vi "frequency_sweep_modulation_freq_smooth.vi"(0 "Frequency":dbl, 1 "Channel (1:Channel 1)":i32, 2 "Amplitude (1.0 Vpp)":dbl=1.0 min=0.001 max=20.0 step=1.0 format="%#.3f", 3 "DC Offset (0.00 V)":dbl min=-10.0 max=10.0, 4 "SG Device 2":T1(ring) caption="Signal Generator Device", 5 "Modulation frequency":dbl[](array[numeric]), 6 "Current Sweep Value":refnum<vi>, 7 "Delay":dbl, 8 "Start t":refnum<vi>, 9 "Modulation Depth (0.0 %)":dbl, 11 "error in (no error)":errorcluster, 12 "Siglent Name":refnum<visa-resource-name>="USB0::0xF4EC::0x1102::SDG2XCAD4R3627::INSTR", 13 "AD2 2":i32, 14 "Stop 2":bool) -> (15 "error out":errorcluster)   [LabVIEW 2024, in "Sweep.lvlib"]
uses:
  Sweep.lvlib
  AD2/Node Parameters.ctl
  <instrlib>/Siglent SDG 1000 5000 800 Series/Public/Configure/Configure Modulation (AM).vi
  <instrlib>/Siglent SDG 1000 5000 800 Series/Siglent SDG 1000 5000 800 Series.lvlib
  AD2/AD2 DLL.lvlib
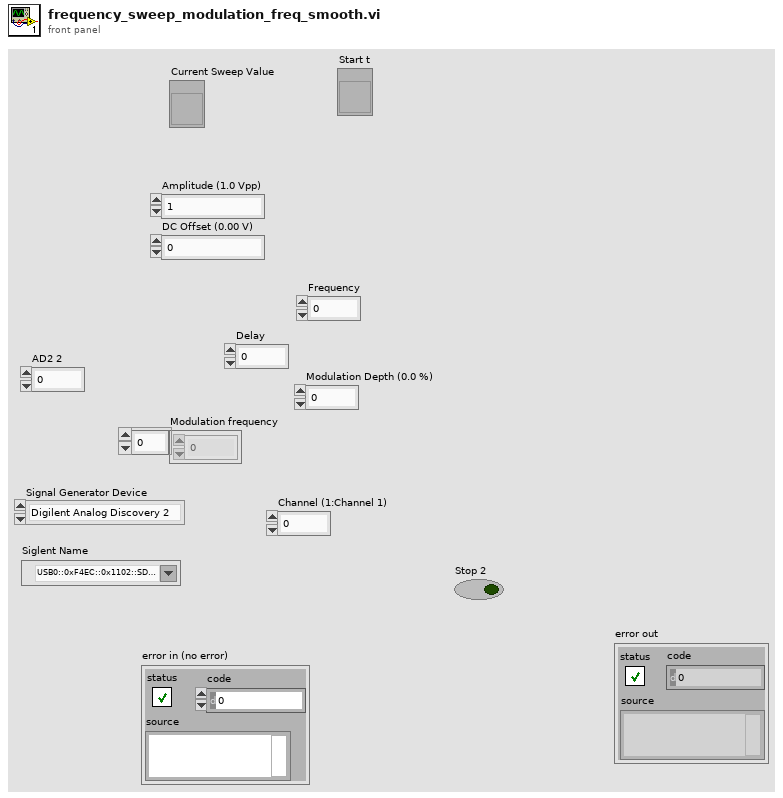
[diagram p1: front panel]
types:
  T1 = enum16{"Digilent Analog Discovery 2", "Siglent DG"}
  T2 = typedef "AD2 DLL.lvlib/Node Parameters.ctl" = cluster{"Function":u8, "Frequency":dbl, "Amplitude":dbl, "DC Offset":dbl, "Duty Cycle":dbl, "Phase":dbl}
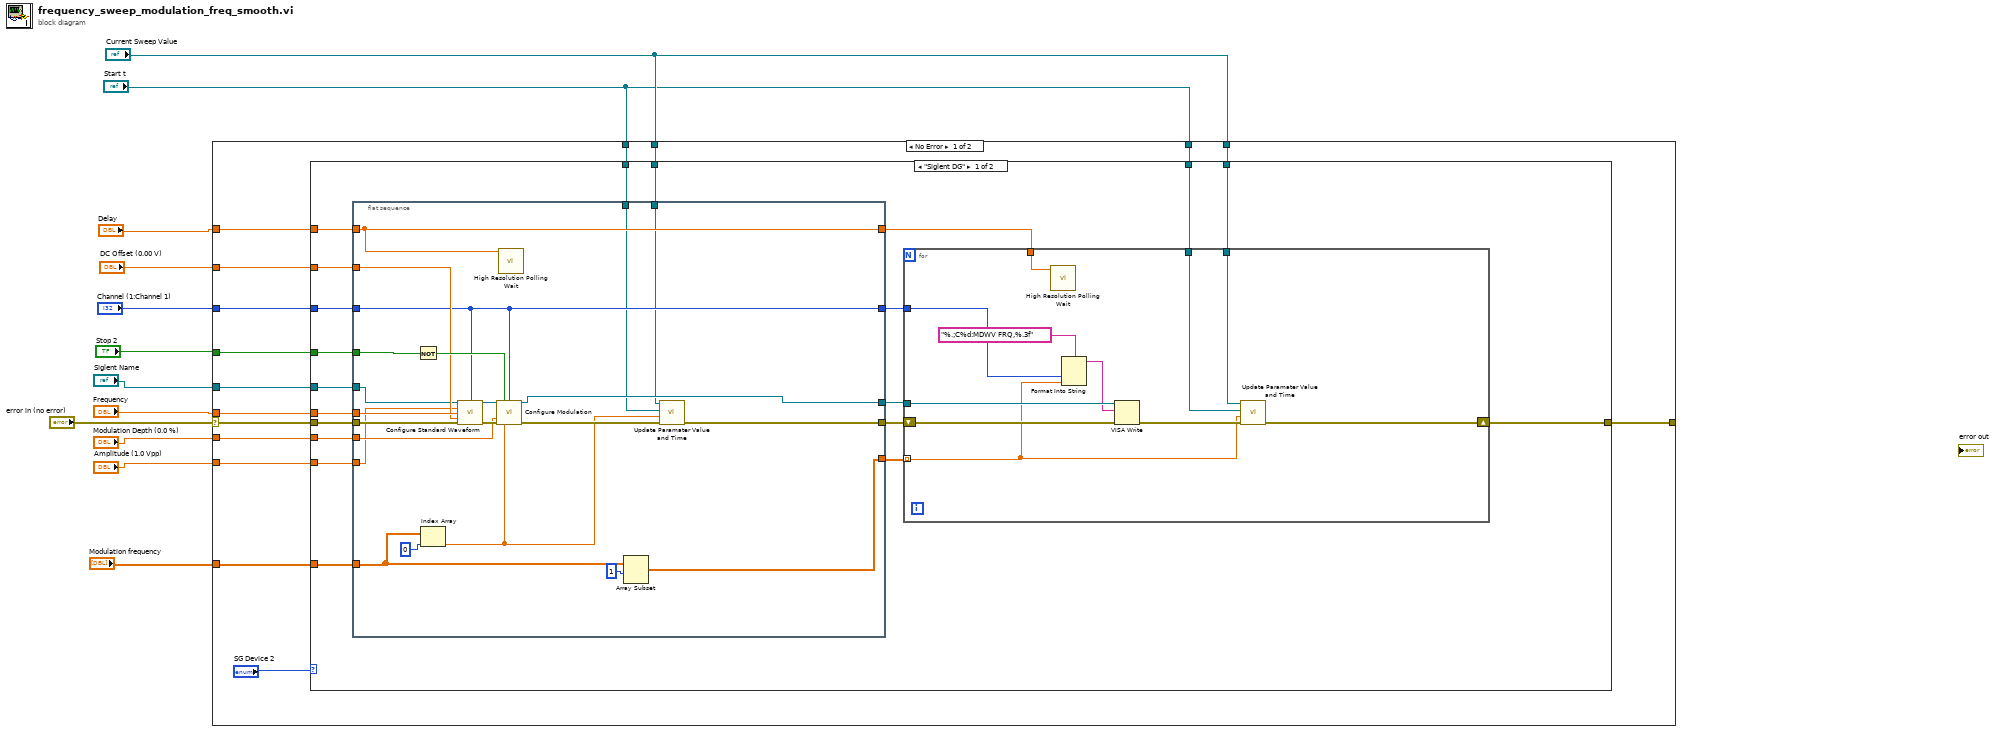
[diagram p0: block diagram]
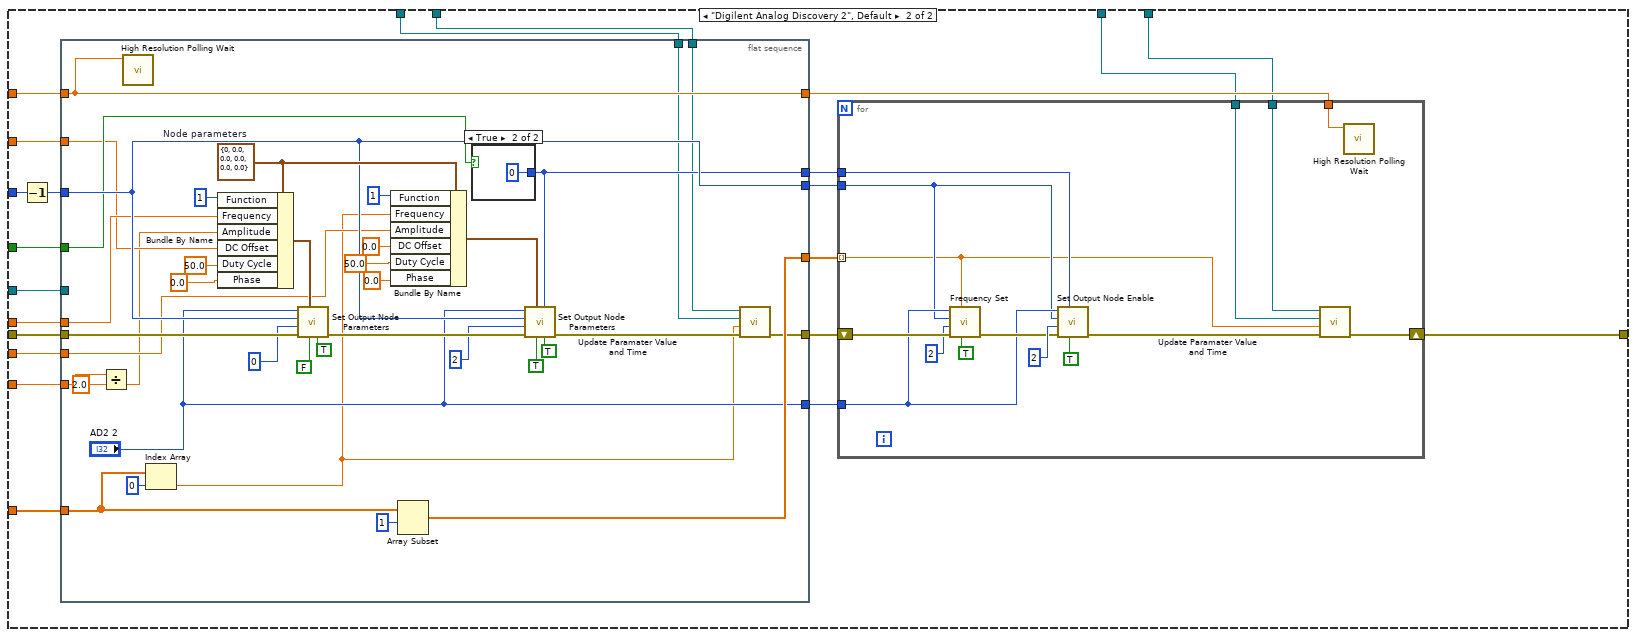
[diagram p2: hidden frame]
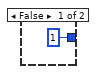
[diagram p3: hidden frame]
diagram:
  n1 = case shown="No Error" "error in (no error)" {
    selector: "error in (no error)" -> [w18 w159]
    tunnel: "Modulation Depth (0.0 %)" -> [w28 _]
    tunnel: "Amplitude (1.0 Vpp)" -> [w27 _]
    tunnel: "Frequency" -> [w26 _]
    tunnel: "Stop 2" -> [w25 _]
    tunnel: [w24 w159] -> _
    tunnel: "Modulation frequency" -> [w23 _]
    tunnel: "Channel (1:Channel 1)" -> [w22 _]
    tunnel: "Delay" -> [w21 _]
    tunnel: "DC Offset (0.00 V)" -> [w20 _]
    tunnel: "Siglent Name" -> [w19 _]
    tunnel: "Current Sweep Value" -> [w16 _]
    tunnel: "Current Sweep Value" -> [w15 _]
    tunnel: "Start t" -> [w14 _]
    tunnel: "Start t" -> [w13 _]
    frame No Error {
      n2 = case shown="\"Siglent DG\"" "SG Device 2" {
        tunnel: w28 -> [w47 w103]
        tunnel: w27 -> [w46 w102]
        tunnel: w26 -> [w45 w101]
        tunnel: w25 -> [w44 w100]
        tunnel: [w42 w98] -> w24
        tunnel: w23 -> [w41 w97]
        tunnel: w22 -> [w39 w95]
        tunnel: w21 -> [w38 w94]
        tunnel: w20 -> [w37 w93]
        tunnel: w19 -> [w36 w92]
        tunnel: w18 -> [w35 w91]
        tunnel: w16 -> [w32 w85]
        tunnel: w15 -> [w31 w84]
        tunnel: w14 -> [w30 w83]
        tunnel: w13 -> [w29 w82]
        frame "Siglent DG" {
          n3 = flat-sequence {
            tunnel: [w69] -> w48
            tunnel: w47 -> [w66]
            tunnel: w46 -> [w54]
            tunnel: w45 -> [w65]
            tunnel: w44 -> [w64]
            tunnel: [w52] -> w43
            tunnel: w41 -> [w62]
            tunnel: [w60] -> w40
            tunnel: w39 -> [w55]
            tunnel: w38 -> [w56]
            tunnel: w37 -> [w59]
            tunnel: w36 -> [w58]
            tunnel: w35 -> [w57]
            tunnel: [w56] -> w34
            tunnel: [w55] -> w33
            tunnel: w32 -> [w49]
            tunnel: w30 -> [w50]
            frame #0 {
              n4 = Not(x=w64) -> (.not. x?=w70:bool)
              n5 = Index Array(array=w62, index=0) -> (element=w51:dbl)
              n6 = call <instrlib>:"Configure Standard Waveform.vi"("VISA resource name"=w58, "Channel (1:Channel 1)"=w55, "Amplitude (1.0 Vpp)"=w54, "Frequency (1000 Hz)"=w65, "DC Offset (0.00 V)"=w59, "error in (no error)"=w57) -> ("VISA resource name out"=w67:refnum<visa-resource-name>, "error out"=w68:errorcluster)  [unwired: 8 in]
              n7 = call-poly <instrlib>:"Configure Modulation.vi"("VISA resource name"=w67, "Enable Amplitude Modulation (T:Enable)"=w70, "Channel (1:Channel 1)"=w55, "Modulation Depth (0.0 %)"=w66, "error in (no error)"=w68, "Modulation Frequency (100 Hz)"=w51) -> ("VISA resource name out"=w69:refnum<visa-resource-name>, "error out"=w53:errorcluster)  [unwired: 8 in]
              n8 = call <vilib>:"High Resolution Polling Wait.vi"("seconds to wait"=w56) -> ()  [unwired: 10 in, 1 out]
              n9 = Array Subset "Array Subset"(array=w62, index=1) -> (w60:dbl[])  [unwired: 1 in]
              n10 = call "Update Paramater Value and Time.vi"("error in (no error)"=w53, "Value"=w51, "Start t"=w50, "Current Sweep Value"=w49) -> ("error out"=w52:errorcluster)  [unwired: 7 in]
            }
          }
          n11 = for {
            shift-right: [w74] -> w42
            shift-left: w43 -> [w77]
            tunnel: w48 -> [w79]
            tunnel: w34 -> [w76]
            tunnel: w40 -> [w73] mode=indexing
            tunnel: w33 -> [w81]
            tunnel: w31 -> [w72]
            tunnel: w29 -> [w71]
            n12 = call <vilib>:"High Resolution Polling Wait.vi"("seconds to wait"=w76) -> ()  [unwired: 10 in, 1 out]
            n13 = Format Into String(format string="%.;C%d:MDWV FRQ,%.3f", w81, w73) -> (resulting string=w78:string)  [unwired: 2 in, 1 out]
            n14 = VISA Write(VISA resource name=w79, write buffer=w78, error in (no error)=w77) -> (error out=w75:errorcluster)  [unwired: 2 out]
            n15 = call "Update Paramater Value and Time.vi"("error in (no error)"=w75, "Value"=w73, "Start t"=w71, "Current Sweep Value"=w72) -> ("error out"=w74:errorcluster)  [unwired: 7 in]
          }
        }
        frame "Digilent Analog Discovery 2", Default {
          n16 = Decrement(x=w95) -> (x-1=w89:i32)
          n17 = flat-sequence {
            tunnel: w103 -> [w119]
            tunnel: w102 -> [w110]
            tunnel: w101 -> [w115]
            tunnel: w100 -> [w120]
            tunnel: [w107] -> w99
            tunnel: w97 -> [w140]
            tunnel: [w138] -> w96
            tunnel: w89 -> [w123]
            tunnel: w94 -> [w137]
            tunnel: w93 -> [w114]
            tunnel: w92 -> [_]
            tunnel: w91 -> [w136]
            tunnel: [w137] -> w86
            tunnel: [w123] -> w90
            tunnel: ["AD2 2"] -> w88
            tunnel: [w113] -> w87
            tunnel: w85 -> [w106]
            tunnel: w83 -> [w105]
            frame #0 {
              w127 = T2 {"Function"=0, "Frequency"=0.0, "Amplitude"=0.0, "DC Offset"=0.0, "Duty Cycle"=0.0, "Phase"=0.0}  # Node parameters
              n18 = Divide(x=w110, y=2.0) -> (x/y=w111:dbl)
              n19 = call <vilib>:"High Resolution Polling Wait.vi"("seconds to wait"=w137) -> ()  [unwired: 10 in, 1 out]
              n20 = Index Array(array=w140, index=0) -> (element=w104:dbl)
              n21 = Bundle By Name(cluster=w127, "Function"=u8 1, "Frequency"=w115, "Amplitude"=w111, "DC Offset"=w114, "Duty Cycle"=50.0, "Phase"=0.0) -> (w134:T2)
              n22 = call "Set Output Node Parameters.vi"("Apply parameters"=TRUE, "Use Enable"=FALSE, "Node parameters"=w134, "error in (no error)"=w136, "node"=0, "idxChannel"=w123, "hdwf"="AD2 2") -> ("error out"=w135:errorcluster)  [unwired: 3 in, 1 out]
              n23 = Bundle By Name(cluster=w127, "Function"=u8 1, "Frequency"=w104, "Amplitude"=w119, "DC Offset"=0.0, "Duty Cycle"=50.0, "Phase"=0.0) -> (w126:T2)
              n24 = Array Subset "Array Subset"(array=w140, index=1) -> (w138:dbl[])  [unwired: 1 in]
              n25 = case shown="True" w120 {
                tunnel: [1 ("Enable") 0 ("Enable")] -> w113
                frame False {
                }
                frame True {
                }
              }
              n26 = call "Set Output Node Parameters.vi"("Apply parameters"=TRUE, "Enable"=w113, "Use Enable"=TRUE, "Node parameters"=w126, "error in (no error)"=w135, "node"=2, "idxChannel"=w123, "hdwf"="AD2 2") -> ("error out"=w108:errorcluster)  [unwired: 2 in, 1 out]
              n27 = call "Update Paramater Value and Time.vi"("error in (no error)"=w108, "Value"=w104, "Start t"=w105, "Current Sweep Value"=w106) -> ("error out"=w107:errorcluster)  [unwired: 7 in]
            }
          }
          n28 = for {
            shift-right: [w147] -> w98
            shift-left: w99 -> [w154]
            tunnel: w96 -> [w144] mode=indexing
            tunnel: w90 -> [w151]
            tunnel: w88 -> [w152]
            tunnel: w87 -> [w157]
            tunnel: w86 -> [w156]
            tunnel: w84 -> [w146]
            tunnel: w82 -> [w145]
            n29 = call "Frequency Set.vi"("Update"=TRUE, "Frequency"=w144, "error in (no error)"=w154, "node"=2, "idxChannel"=w151, "hdwf"=w152) -> ("error out"=w153:errorcluster)  [unwired: 3 in, 2 out]
            n30 = call "Set Output Node Enable.vi"("Update"=TRUE, "Enable"=w157, "error in (no error)"=w153, "node"=2, "idxChannel"=w151, "hdwf"=w152) -> ("error out"=w148:errorcluster)  [unwired: 4 in, 1 out]
            n31 = call "Update Paramater Value and Time.vi"("error in (no error)"=w148, "Value"=w144, "Start t"=w145, "Current Sweep Value"=w146) -> ("error out"=w147:errorcluster)  [unwired: 7 in]
            n32 = call <vilib>:"High Resolution Polling Wait.vi"("seconds to wait"=w156) -> ()  [unwired: 10 in, 1 out]
          }
        }
      }
    }
    frame Error {
    }
  }
